vi "Tiempo_Rampa.vi"(0 "Start_A":dbl caption="Ángulo inicial" min=-5.0 max=5.0 step=0.05, 1 "Stop_A":dbl caption="Ángulo final" min=-5.0 max=5.0 step=0.05, 2 "Step_A":dbl=0.01 caption="Paso ángulo" min=0.01 max=1.0 step=0.01, 3 "ms to wait":u32=7 min=7 max=1000 step=1, 5 "Error In":errorcluster) -> (14 "Time_Rampa":dbl, 19 "Error Out":errorcluster)   [LabVIEW 2016]
doc: "Calcula el tiempo que toma una rampa"
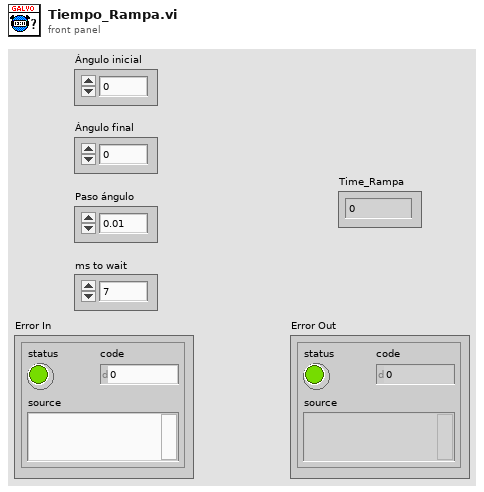
[diagram p1: front panel]
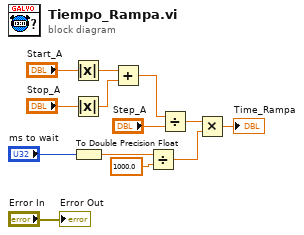
[diagram p0: block diagram]
diagram:
  n1 = Absolute Value(x="Start_A") -> (abs(x)=w11:dbl)
  n2 = Absolute Value(x="Stop_A") -> (abs(x)=w10:dbl)
  n3 = To Double Precision Float(number="ms to wait") -> (double precision float=w4:dbl)
  n4 = Add(x=w11, y=w10) -> (x+y=w9:dbl)
  n5 = Divide(x=w4, y=1000.0) -> (x/y=w1:dbl)
  n6 = Divide(x=w9, y="Step_A") -> (x/y=w7:dbl)
  n7 = Multiply(x=w7, y=w1) -> (x*y=→"Time_Rampa":dbl)
  "Error Out" <- "Error In"
